vi "Robot Systems.vi"(11 "input cluster":T1) -> ()   [LabVIEW 2015]
uses:
  Joystick/ControlsToCommands.ctl
panel:
  out "Temporary Center":dbl
  out "Stuck?":bool
  out "Position":dbl
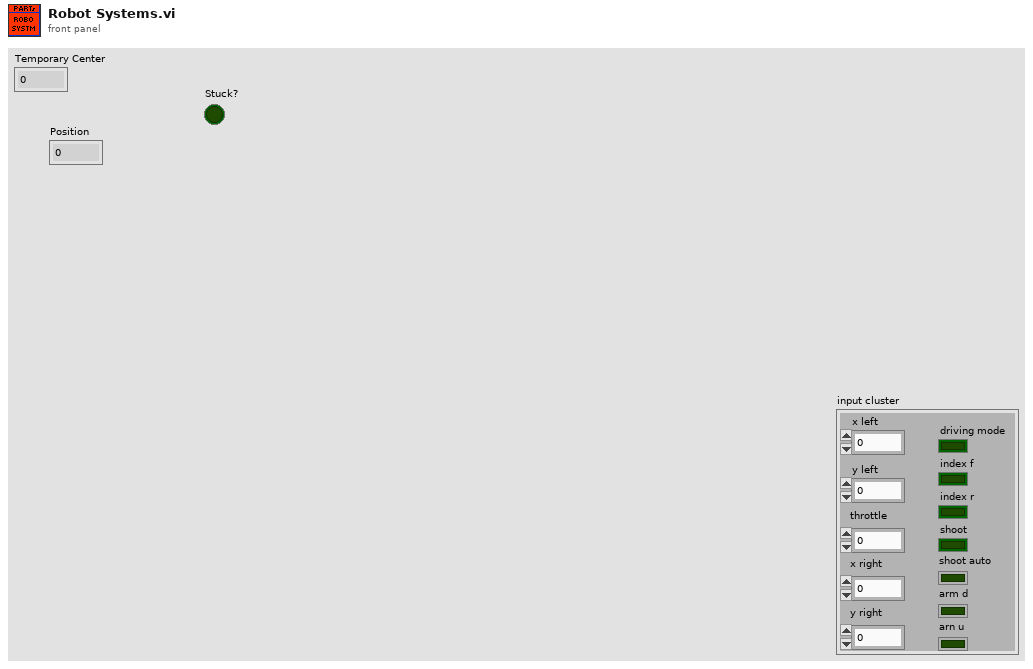
[diagram p1: front panel]
types:
  T1 = typedef "ControlsToCommands.ctl" = cluster{"x left":dbl, "y left":dbl, "throttle":dbl, "x right":dbl, "y right":dbl, "driving mode":bool, "index f":bool, "index r":bool, "shoot":bool, "shoot auto":bool, "arm d":bool, "arn u":bool}
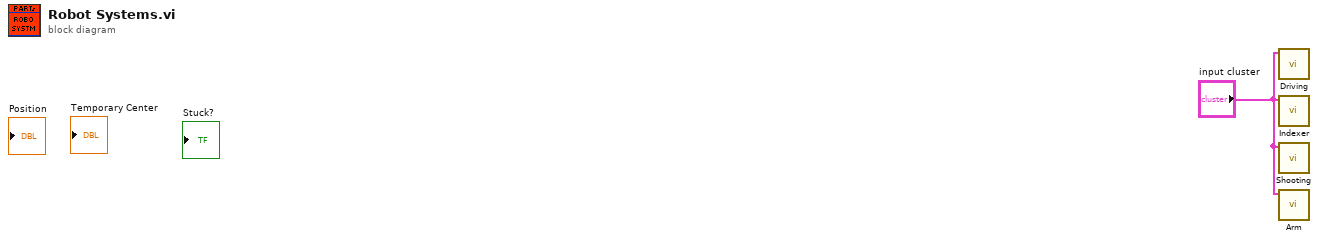
[diagram p0: block diagram]
diagram:
  n1 = call "Driving.vi"("input cluster"="input cluster") -> ()  [unwired: 11 in]
  n2 = call "Indexer.vi"("input cluster"="input cluster") -> ()  [unwired: 11 in]
  n3 = call "Shooting.vi"("input cluster"="input cluster") -> ()  [unwired: 11 in]
  n4 = call "Arm.vi"("input cluster"="input cluster") -> ()  [unwired: 11 in]
